vi "AgilentSweep.vi"(0 "Enable Output (T: Enable)":bool, 1 "IH setgs":T1={"Start Frequency"=12000.0, "Stop Frequency"=15000.0, "Sweep Time"=0.011, "Amplitude"=0.2} {"Sweep Time" format="%.4f"; "Stop Frequency" format="%^.5e"; "Start Frequency" format="%^.5e"; "Amplitude" min=0.0 max=4.0 format="%.3f"}, 2 "VISA resource name":refnum<visa-resource-name>="agi33522a") -> ()   [LabVIEW 2018]
doc: "This example shows how to generate a standard waveform."
uses:
  <instrlib>/Agilent 3352X Series/Agilent 3352X Series.lvlib
panel:
  out "duration (ms)":u32=75
  in  "fstart (Hz)":dbl=12000.0 format="%_4p"
  in  "fstop (Hz)":dbl=15000.0 format="%_4p"
  in  "Amplitude":dbl=0.2
  in  "Channel (1: 1)":i32(ring)=1 items=["1"=1, "2"=2]
  in  "Sweep time (s)":dbl=0.011 format="%_4p"
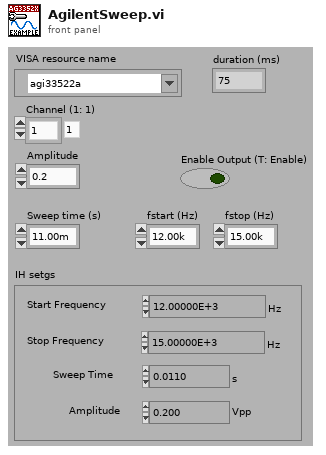
[diagram p1: front panel]
types:
  T1 = cluster{"Start Frequency":dbl, "Stop Frequency":dbl, "Sweep Time":dbl, "Amplitude":dbl}
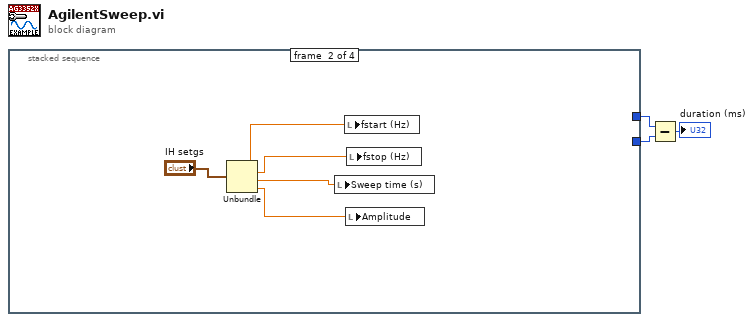
[diagram p0: block diagram]
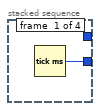
[diagram p2: hidden frame]
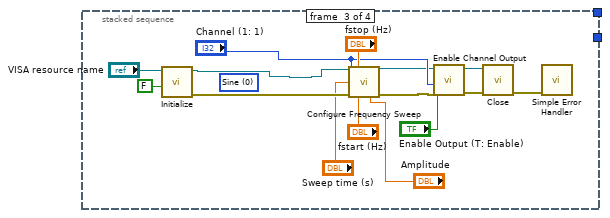
[diagram p3: hidden frame]
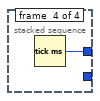
[diagram p4: hidden frame]
diagram:
  n1 = stacked-sequence {
    tunnel: [_ _ _ w25] -> w2
    tunnel: [w4 _ _ _] -> w3
    frame #0 {
      n2 = Tick Count (ms)() -> (millisecond timer value=w4:u32)
    }
    frame #1 {
      n3 = Unbundle("IH setgs") -> ("Start Frequency"=w6:dbl, "Stop Frequency"=w7:dbl, "Sweep Time"=w8:dbl, "Amplitude"=w5:dbl)
      n4 = local write "Sweep time (s)"(w8) -> ()
      n5 = local write "fstart (Hz)"(w6) -> ()
      n6 = local write "Amplitude"(w5) -> ()
      n7 = local write "fstop (Hz)"(w7) -> ()
    }
    frame #2 {
      (unwired) 0 items=["Sine"=0, "Square"=1, "Ramp"=2, "Noise"=3, "DC"=4, "Triangle"=5, "Pulse"=6, "Sinc"=11, "D-Lorentz"=12, "Gaussian"=13, "Expo Fall"=14, "Expo Rise"=15, "Haversine"=16] ("Waveform Function (0: Sine)")
      n8 = call <instrlib>:"Initialize.vi"("Reset (Enable)"=FALSE, "VISA resource name"="VISA resource name") -> ("error out"=w23:errorcluster, "VISA resource name out"=w24:refnum<visa-resource-name>)  [unwired: 3 in, 5 out]
      n9 = call <instrlib>:"Configure Frequency Sweep.vi"("VISA resource name"=w24, "Stop  Frequency (1000 Hz)"="fstop (Hz)", "Sweep Time (1 s)"="Sweep time (s)", "Channel (1: 1)"="Channel (1: 1)", "error in (no error)"=w23, "Start Frequency (100 Hz)"="fstart (Hz)", "Amplitude (1 Vpp)"="Amplitude") -> ("VISA resource name out"=w16:refnum<visa-resource-name>, "error out"=w15:errorcluster)  [unwired: 7 in]
      n10 = call <instrlib>:"Enable Channel Output.vi"("error in (no error)"=w15, "Channel (1: 1)"="Channel (1: 1)", "Enable Output (T: Enable)"="Enable Output (T: Enable)", "VISA resource name"=w16) -> ("error out"=w12:errorcluster, "VISA resource name out"=w13:refnum<visa-resource-name>)  [unwired: 6 in]
      n11 = call <instrlib>:"Close.vi"("error in (no error)"=w12, "VISA resource name"=w13) -> ("error out"=w22:errorcluster)  [unwired: 9 out]
      n12 = call <vilib>:"Simple Error Handler.vi"("error in (no error)"=w22) -> ()  [unwired: 1 in, 8 out]
    }
    frame #3 {
      n13 = Tick Count (ms)() -> (millisecond timer value=w25:u32)
    }
  }
  n14 = Subtract(x=w2, y=w3) -> (x-y=→"duration (ms)":u32)
